vi "UI_Elmt_Read(Label).vi"(8 "error in (no error)":errorcluster, 10 "Elmt Label":string, 11 "UI_Actor in":refnum<class "UI_Actor.lvclass">) -> (0 "error out":errorcluster, 1 "Found":bool, 2 "Value":variant, 3 "UI_Actor out":refnum<class "UI_Actor.lvclass">)   [LabVIEW 2020, in "UI_Actor.lvlib" / "UI_Actor.lvclass"]
doc: "Accès à un élément par son label.\n<b> NEVER USE IN FOR LOOP </b> \nLa ref est stockée au premier appel en fgv.\nLe VI doit etre dédié à un unique élement."
uses:
  UI_Actor.lvclass
  UI_Actor.lvclass/UI_Actor.ctl
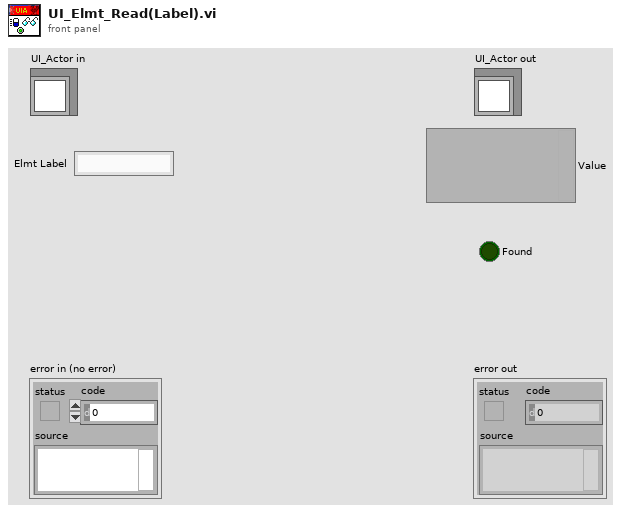
[diagram p1: front panel]
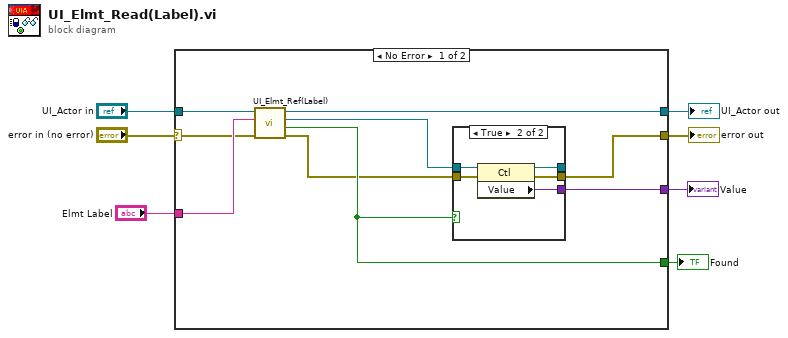
[diagram p0: block diagram]
diagram:
  n1 = case shown="No Error" "error in (no error)" {
    selector: "error in (no error)" -> [w9 w25]
    tunnel: [w15 w25] -> w6
    tunnel: [w11 w24] -> w4
    tunnel: "UI_Actor in" -> [w10 w24]
    tunnel: "Elmt Label" -> [w16 _]
    tunnel: [w14 _] -> w2
    tunnel: [w12 _] -> w1
    frame No Error {
      n2 = call "UI_Elmt_Ref(Label).vi"("error in (no error)"=w9, "Elmt Label"=w16, "UI_Actor in"=w10) -> ("error out"=w8:errorcluster, "Found"=w12:bool, "Ctl Refnum"=w13:refnum<vi>, "UI_Actor out"=w11:refnum<class "UI_Actor.lvclass">)  [unwired: 5 in]
      n3 = case shown="True" w12 {
        tunnel: w8 -> [w17 w23]
        tunnel: [w17 w22] -> w15
        tunnel: w13 -> [w18 w21]
        tunnel: [_ w20] -> w14
        tunnel: [w18 w19] -> _
        frame False {
        }
        frame True {
          n4 = property class="Ctl"(reference=w21, error in=w23) -> (reference out=w19:refnum<vi>, error out=w22:errorcluster, "Value"=w20:variant)
        }
      }
    }
    frame Error {
    }
  }
  "error out" <- w6
  "UI_Actor out" <- w4
  "Value" <- w2
  "Found" <- w1
